vi "caps.vi"() -> ()   [LabVIEW 2015]
panel:
  in  "String 2":string
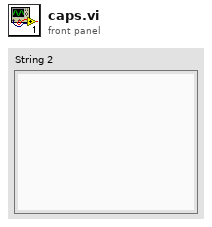
[diagram p1: front panel]
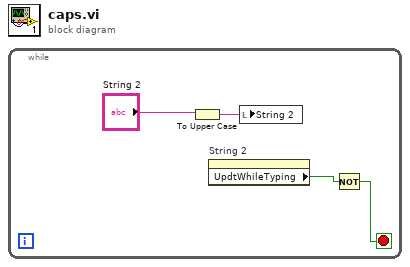
[diagram p0: block diagram]
diagram:
  n1 = while {
    stop <- w1 stop-if-true
    n2 = To Upper Case(1:"String 2") -> (0:w3:string)
    n3 = property on="String 2" class="Str"() -> ("UpdtWhileTyping"=w2:bool)  [unwired: 2 in, 2 out]
    n4 = local write "String 2"(w3) -> ()
    n5 = Not(x=w2) -> (.not. x?=w1:bool)
  }
